vi "Save Digital Data.vi"(8 "error in (no error)":errorcluster, 10 "Data Cluster":cluster{"Path":path, "Array":bool[]}, 11 "Digital Plain Text in":refnum<class "Digital Plain Text.lvclass">) -> (0 "error out":errorcluster, 3 "Digital Plain Text out":refnum<class "Digital Plain Text.lvclass">)   [LabVIEW 2020, in "Digital Plain Text.lvlib" / "Digital Plain Text.lvclass"]
uses:
  Digital Plain Text.lvclass
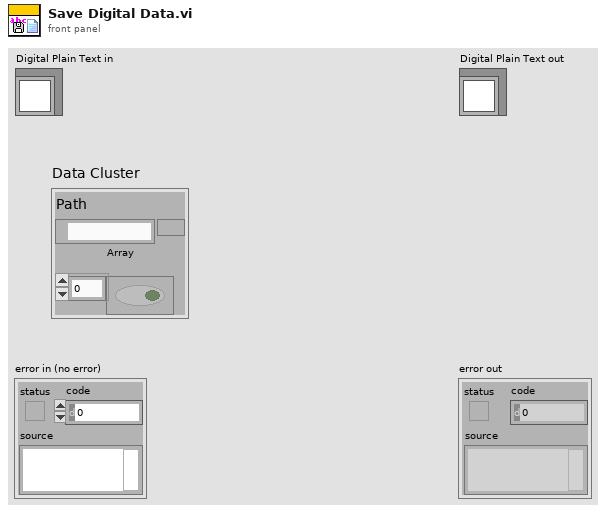
[diagram p1: front panel]
types:
  T1 = enum16{"open", "replace", "create", "open or create", "replace or create", "replace or create with confirmation"}
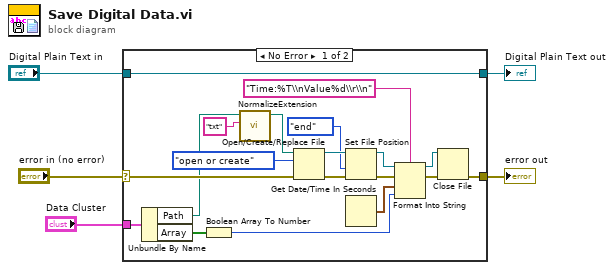
[diagram p0: block diagram]
diagram:
  n1 = case shown="No Error" "error in (no error)" {
    selector: "error in (no error)" -> [w21 w26]
    tunnel: [w13 w26] -> w4
    tunnel: "Digital Plain Text in" -> [w24 w25]
    tunnel: [w24 w25] -> w2
    tunnel: "Data Cluster" -> [w23 _]
    frame No Error {
      n2 = Unbundle By Name(w23) -> ("Path"=w6:path, "Array"=w22:bool[])
      n3 = Boolean Array To Number(Boolean array=w22) -> (number=w9:u32)
      n4 = call "NormalizeExtension.vi"("Extension"="txt", "Path in"=w6) -> ("Path out"=w19:path)  [unwired: 9 in]
      n5 = Open/Create/Replace File(file path (use dialog)=w19, error in=w21, operation (0:open)=T1."open or create") -> (refnum out=w16:refnum<file>, error out=w17:errorcluster)  [unwired: 3 in, 1 out]
      n6 = Set File Position(refnum=w16, from (0:start)=enum16{"start", "end", "current"}."end", error in=w17) -> (refnum out=w7:refnum<file>, error out=w12:errorcluster)  [unwired: 1 in]
      n7 = Get Date/Time In Seconds() -> (seconds since 1Jan1904=w10:timestamp)
      n8 = Format Into String(format string="Time:%T\\nValue%d\\r\\n", initial string=w7, error in=w12, w10, w9) -> (resulting string=w14:refnum<file>, error out=w15:errorcluster)
      n9 = Close File(refnum=w14, error in=w15) -> (error out=w13:errorcluster)  [unwired: 1 out]
    }
    frame Error {
    }
  }
  "error out" <- w4
  "Digital Plain Text out" <- w2
